vi "Modulo_Triggers.vi"(0 "Motion Settings In":T1={"No Motion?"=FALSE, "Motion System"=enum."NI 735x", "Motion Bd ID"=1, "Motion Profile"="SMAC1", "# Axis"=1, "Reverse Z axis?"=TRUE, "SMAC Axis"=0, "scan pair"=enum."y-(x) scan", "RT fps"=6.0, "Steps per mm"=[1000, 1000, 1000, 1000], "Motor Parameters"={"velocity ct/s"=[10000.0, 10000.0, 10000.0, 50000.0], "accel ct/s^2"=[50000.0, 50000.0, 50000.0, 200000.0]}, "One Way Scan"=FALSE, "Reverse One Way Scan"=FALSE, "Global Position (mm)"=[], "Plane"=0, "Distance between\nscan lines (um)"=0.0, "Distance between\nscan planes (um)"=0.0, "number of scan planes"=1, "Total steps in line"=0, "Xtra plane\ndistance  (um)"=100, "Xtra planes "=1, "Add Axis"=FALSE, "overshoot cts"=200, "BKPT Shift"=0, "Scan Start Time (ms)"=0, "ESP VISA"="GPIB::1::INSTR", "3rd Axis"=1, "GL Ref Out"=refnum, "Galil Address"=""} {"3rd Axis" items=["x", "y", "z", "w"]; "Xtra planes" min=1; "Xtra plane\ndistance  (um)" min=0; "Distance between\nscan planes (um)" format="%.2f"; "Distance between\nscan lines (um)" format="%.2f"; "SMAC Axis" items=["None"=0, "Axis 1"=1, "Axis 2"=2, "Axis 3"=3, "Axis 4"=4, "Axis 5"=5, "Axis 6"=6, "Axis 7"=7, "Axis 8"=8, "Vector Space 1"=17, "Vector Space 2"=18, "Vector Space 3"=19, "Vector Space 4"=20]; "Motion Bd ID" min=1 max=32 step=1}, 1 "Axis":u16(ring)=1 items=["Axis 1"=1, "Axis 2"=2, "Axis 3"=3, "Axis 4"=4, "Axis 5"=5, "Axis 6"=6, "Axis 7"=7, "Axis 8"=8], 2 "Reverse ?":bool, 5 "Program (1)":u8=4 format="%.0x", 11 "error in (no error)":errorcluster, 13 "Offset":i32) -> (4 "Start Position":i32, 15 "error out":errorcluster)   [LabVIEW 2022 SP3]
doc: "EXAMPLE: DO_WHILE Loop (Onboard Programming Template)\n\nSUMMARY:\nThis FlexMotion example demonstrates the implementation of a DO_WHILE loop data structure in an onboard program. The C equivalent of the data structure implemented here is:\n\ndo {\n// code to be repeated\nloopVar = loopVar - increment;\n} while (loopVar != 0);\n\nTHEORY OF OPERATION:\nThe flow of the DO_WHILE loop data structure goes as follows:\n(1) Program storage is begun.\n(2) The DO_WHILE loop is set up. (Loop Variable and Increment are each defined and initialized.)\n(3) A code delimiter is set using label #1.\n(4) Code to be executed each time through loop is run (in the template program, the loop variable is decremented).\n(5) The loop variable or other test condition is checked.\n(6) If the test condition is true, then we jump back to label #1. Otherwise, the condition is false so the loop terminates.\n(7) Program storage is ended.\n\nDEVELOPMENT DETAILS:\nApplication Software: LabVIEW 5.0.x\nHardware: FlexMotion controller\nDriver Software: FlexMotion Software 4.0\n\nREQUIRED HARDWARE:\n(controller only)\n\nINSTRUCTIONS:\n(0) Initialize the FlexMotion controller before running this VI. \n(1) Add the FlexMotion functions you want to execute into the block diagram where noted.\n(2) Run the VI to store the program. (The program will not be executed at this time.)\n(3) You can then run the program you have stored by calling the run_prog.flx function with the appropriate program number.\n\nADDITIONAL NOTES:\n(a) You should read the following items before writing FlexMotion onboard programs:\n(1) The Onboard Programs section of the FlexMotion Hardware User Manual (page 4-9 in the November 1998 edition).\n(2) The section about onboard variables in your FlexMotion Software Reference Manual (pages 4-11 and 4-12 in the November 1998 edition)\n(3) You will find the chapter of the FlexMotion Software Reference Manual concerning the Onboard Programming functions to be an invaluable reference resource (Chapter 12 of the November 1998 edition) along with the online help for the VI functions.\n(b) This template repeats the DO_WHILE loop as long as an expression with a variable evaluates to be true. However, you may evaluate other conditions such as move complete status instead.\n\n*NOTE: This example is not supported on the 7334 controller."
uses:
  MotionParameters.ctl
  MotionSys.ctl
  -MotionRoutines/ScanAxis.ctl
  -MotionRoutines/3rdAxis.ctl
  <vilib>/Motion/FlexMotion/FunctionsVIs/StartStopMotion.llb/Start Motion (8 axes).flx
  <vilib>/Motion/FlexMotion/FunctionsVIs/Trajectory.llb/Load Acceleration/Deceleration.flx
  <vilib>/Motion/FlexMotion/FunctionsVIs/OnboardProgramming.llb/Jump to Label on Condition (8 axes).flx
  <vilib>/Motion/FlexMotion/FunctionsVIs/OnboardProgramming.llb/Wait on Condition (8 axes).flx
panel:
  out "Store Loop":i32
  # "This will only work with735X controllers"
  # "1-D and 2-D B scan settings"
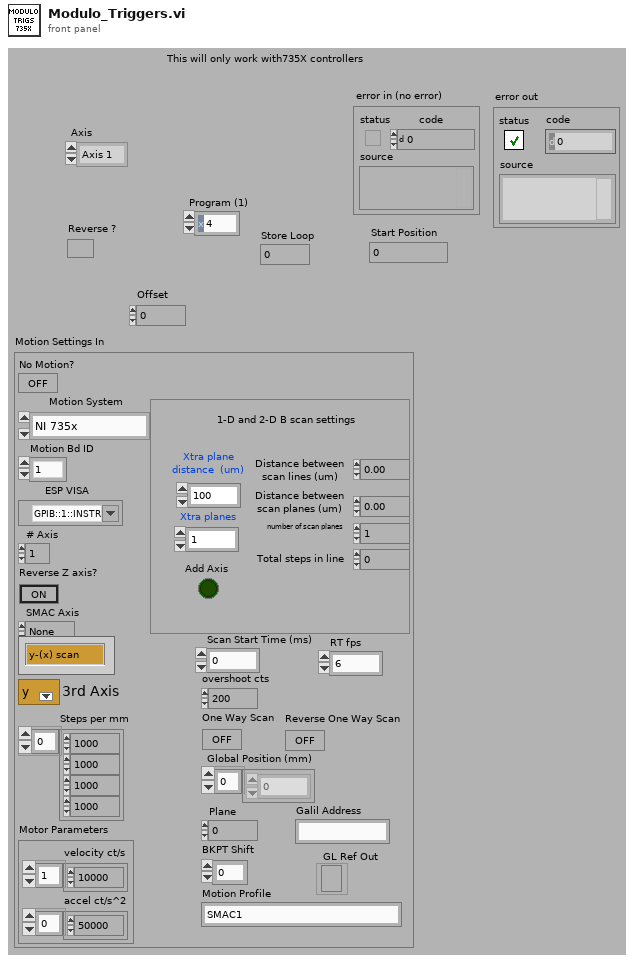
[diagram p1: front panel]
types:
  T1 = typedef "MotionParameters.ctl" = cluster{"No Motion?":bool, "Motion System":T2, "Motion Bd ID":u8, "Motion Profile":string, "# Axis":i8, "Reverse Z axis?":bool, "SMAC Axis":u16, "scan pair":T3, "RT fps":sgl, "Steps per mm":i32[], "Motor Parameters":cluster{"velocity ct/s":dbl[], "accel ct/s^2":dbl[]}, "One Way Scan":bool, "Reverse One Way Scan":bool, "Global Position (mm)":dbl[], "Plane":i32, "Distance between\nscan lines (um)":sgl, "Distance between\nscan planes (um)":sgl, "number of scan planes":i32, "Total steps in line":i32, "Xtra plane\ndistance  (um)":i32, "Xtra planes ":i32, "Add Axis":bool, "overshoot cts":i32, "BKPT Shift":i32, "Scan Start Time (ms)":u32, "ESP VISA":refnum<visa-resource-name>, "3rd Axis":T4, "GL Ref Out":refnum<k7>, "Galil Address":string}
  T2 = typedef "MotionSys.ctl" = enum16{"MM3000", "NI 735x", "Newport ESP", "No Motion Card", "Galil"}
  T3 = typedef "ScanAxis.ctl" = enum16{"y-(x) scan", "x-(y) scan", "z-(x) scan", "z-(y) scan", "y-(z) scan", "x-(z) scan", "w-(x) scan", "w-(y) scan", "w-(z) scan", "x-(w) scan", "y-(w) scan", "z-(w) scan"}
  T4 = typedef "3rdAxis.ctl" = u16
  T5 = enum16{"No Change", "Reset on Breakpoint", "Set on Breakpoint", "Toggle on Breakpoint", "Create Pulse on Breakpoint"}
  T6 = enum16{"Absolute Breakpoint", "Relative Breakpoint", "Modulo Breakpoint", "Periodic Breakpoint"}
  T7 = typedef "Var" = u8
  T8 = enum16{"Less Than", "Equal", "Less Than Or Equal", "Greater Than", "Not Equal", "Greater Than Or Equal", "True", "Home Found", "Index Found", "High Speed Capture", "Position Breakpoint", "Reserved", "Velocity Threshold", "Move Complete", "Profile Complete", "Blend Complete", "Motor Off", "Home Input Active", "Limit Input Active", "Software Limit Active", "Program Complete", "IO Port Match"}
  T9 = typedef "Bd Id Out" = u8
  T10 = typedef "Resource Out (Enum).flx" = u16
  T11 = typedef "Resource Out.flx" = u8
  T12 = cluster{"0":bool, "1":bool, "2":bool, "3":bool, "4":bool, "5":bool, "6":bool, "7":bool, "8":bool}
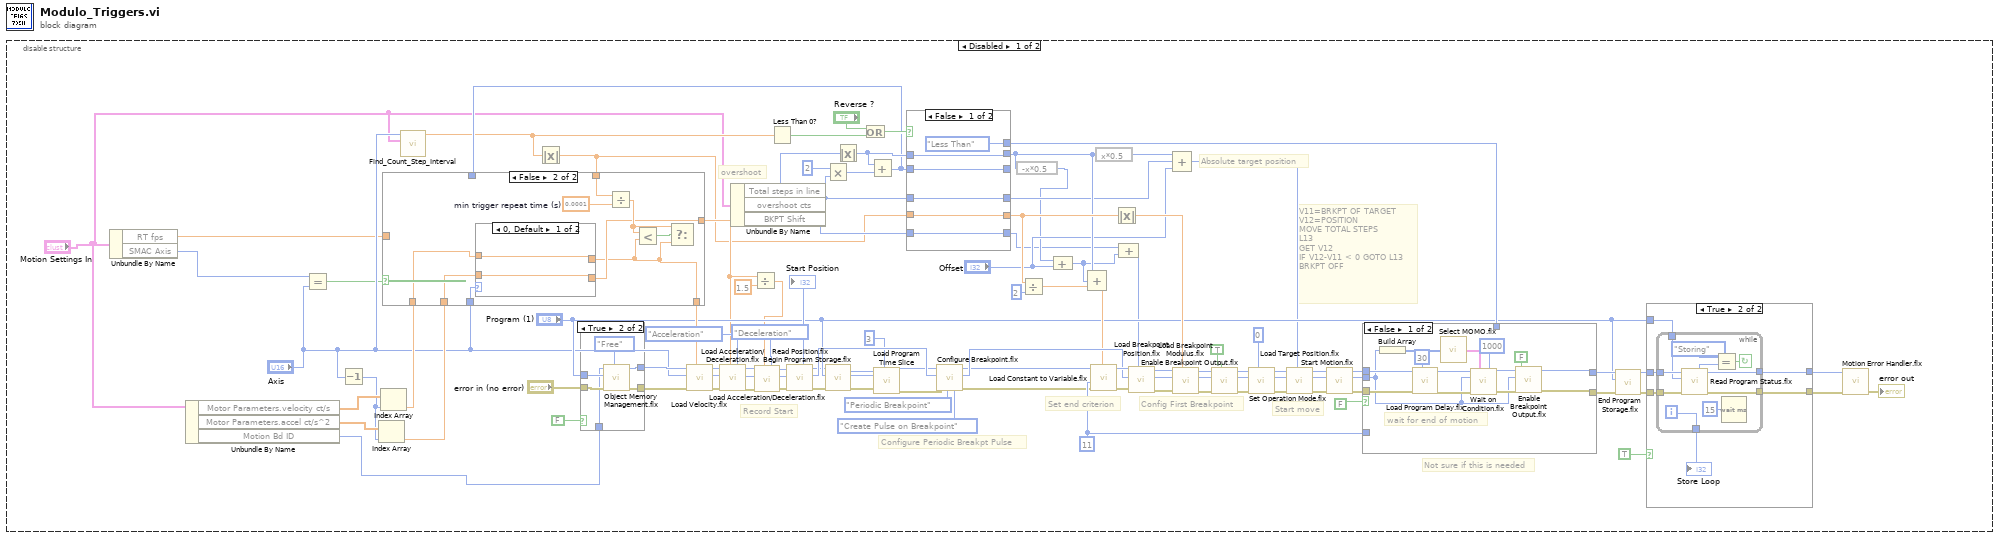
[diagram p0: block diagram]
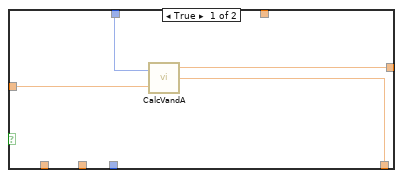
[diagram p4: hidden frame]
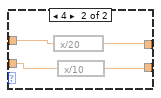
[diagram p5: hidden frame]
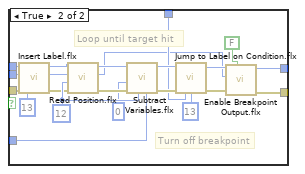
[diagram p6: hidden frame]
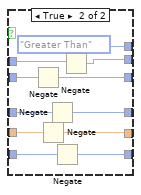
[diagram p7: hidden frame]
diagram:
  n1 = disable-structure shown="Disabled" {
    frame Disabled {
      w105 = T7 11 ("Step Int Variable")
      # "Absolute target position"
      # "Not sure if this is needed"
      # "Configure Periodic Breakpt Pulse"
      # "Set end criterion"
      # "overshoot"
      # "V11=BRKPT OF TARGET\nV12=POSITION\nMOVE TOTAL STEPS\nL13\nGET V12\nIF V12-V11 < 0 GOTO L13\nBRKPT OFF"
      # "Record Start"
      # "Config First Breakpoint"
      # "Start move"
      n2 = Unbundle By Name("Motion Settings In") -> ("RT fps"=w6:sgl, "SMAC Axis"=w9:u16)
      n3 = Unbundle By Name("Motion Settings In") -> ("Motor Parameters.velocity ct/s"=w16:dbl[], "Motor Parameters.accel ct/s^2"=w15:dbl[], "Motion Bd ID"=w1:u8)
      n4 = Equal?(x=w9, y="Axis") -> (x = y?=w2:bool)
      n5 = Decrement(x="Axis") -> (x-1=w11:u16)
      n6 = Index Array(array=w15, index=w11) -> (element=w13:dbl)
      n7 = Index Array(array=w16, index=w11) -> (element=w14:dbl)
      n8 = call "Find_Count_Step_Interval.vi"("Motion Settings In"="Motion Settings In", "Axis"="Axis") -> ("BP Interval"=w12:dbl)  [unwired: 8 in, 1 out]
      n9 = Absolute Value(x=w12) -> (abs(x)=w3:dbl)
      n10 = case shown="True" FALSE {
        tunnel: "error in (no error)" -> [w107 w112]
        tunnel: "Program (1)" -> [_ w111]
        tunnel: [w106 w110] -> w44
        tunnel: [w107 w109] -> w43
        tunnel: w1 -> [w106 w108]
        frame False {
        }
        frame True {
          n11 = call <vilib>:"Object Memory Management.flx"("Operation"=enum16{"Save", "Delete", "Free"}."Free" ("Operation (Free)"), "error in (no error)"=w112, "Object (1)"=w111, "Board ID"=w108) -> ("error out"=w109:errorcluster, "Bd ID Out"=w110:T9)  [unwired: 4 out]
        }
      }
      n12 = Unbundle By Name("Motion Settings In") -> ("Total steps in line"=w5:i32, "overshoot cts"=w7:i32, "BKPT Shift"=w4:i32)
      n13 = Less Than 0?(x=w12) -> (x < 0?=w94:bool)
      n14 = Multiply(x=2, y=w7) -> (x*y=w58:i32)
      n15 = Absolute Value(x=w5) -> (abs(x)=w64:i32)
      n16 = Or(x="Reverse ?", y=w94) -> (x .or. y?=w92:bool)
      n17 = Add(x=w64, y=w58) -> (x+y=w57:i32)
      n18 = case shown="False" w2 {
        tunnel: [w132 w140] -> w27
        tunnel: [w133 w136] -> w80
        tunnel: w3 -> [_ w141]
        tunnel: w57 -> [w135 _]
        tunnel: w6 -> [w134 _]
        tunnel: "Axis" -> [_ w139]
        tunnel: w14 -> [_ w138]
        tunnel: w13 -> [_ w137]
        frame True {
          n19 = call "CalcVandA.vi"("distance"=w135, "fps"=w134) -> ("Accel"=w132:dbl, "Velocity"=w133:dbl)  [unwired: 1 out]
        }
        frame False {
          w142 = 0.0001  # min trigger repeat time (s)
          n20 = case shown="0, Default" w139 {
            tunnel: w138 -> [w146 w150]
            tunnel: w137 -> [w145 w147]
            tunnel: [w146 w149] -> w136
            tunnel: [w145 w148] -> w140
            frame 0, Default {
            }
            frame 4 {
              n21 = expression code="x/20"(w150) -> (w149:dbl)
              n22 = expression code="x/10"(w147) -> (w148:dbl)
            }
          }
          n23 = Divide(x=w141, y=w142) -> (x/y=w143:dbl)
          n24 = Less?(x=w143, y=w136) -> (x < y?=w144:bool)
          n25 = Select(t=w143, s=w144, f=w136) -> ()  [unwired: 1 out]
        }
      }
      n26 = call <vilib>:"Load Velocity.flx"("Velocity (10000)"=w80, "error in (no error)"=w43, "Axis or Vector Space"="Axis", "Board ID"=w44) -> ("error out"=w91:errorcluster, "Resource Output"=w89:T10, "Bd ID Out"=w90:T9)  [unwired: 3 out]
      n27 = call "Load Acceleration/Deceleration.flx"("Acceleration Type (Both)"=enum16{"Both", "Acceleration", "Deceleration"}."Acceleration", "Acceleration (100000)"=w27, "error in (no error)"=w91, "Axis or Vector Space"=w89, "Board ID"=w90) -> ("error out"=w32:errorcluster, "Resource Output"=w31:T10, "Bd ID Out"=w35:T9)  [unwired: 2 out]
      n28 = Divide(x=w27, y=1.5) -> (x/y=w26:dbl)
      n29 = call "Load Acceleration/Deceleration.flx"("Acceleration Type (Both)"=enum16{"Both", "Acceleration", "Deceleration"}."Deceleration", "Acceleration (100000)"=w26, "error in (no error)"=w32, "Axis or Vector Space"=w31, "Board ID"=w35) -> ("error out"=w33:errorcluster, "Resource Output"=w30:T10, "Bd ID Out"=w34:T9)  [unwired: 2 out]
      n30 = call <vilib>:"Read Position.flx"("error in (no error)"=w33, "Axis"=w30, "Board ID"=w34) -> ("error out"=w52:errorcluster, "Resource Output"=w65:T10, "Bd ID Out"=w53:T9, "Position"=→"Start Position":i32)  [unwired: 3 out]
      n31 = call <vilib>:"Begin Program Storage.flx"("error in (no error)"=w52, "Program (1)"="Program (1)", "Board ID"=w53) -> ("error out"=w42:errorcluster, "Resource Out"=w37:T11, "Bd ID Out"=w39:T9)  [unwired: 3 out]
      n32 = call <vilib>:"Load Program Time Slice.vi"("Time Slice (ms)"=u32 3, "error in (no error)"=w42, "Program"=w37, "Board ID"=w39) -> ("error out"=w41:errorcluster, "Bd ID Out"=w40:T9)  [unwired: 1 in, 2 out]
      n33 = case shown="False" w92 {
        tunnel: w57 -> [w191 w202]
        tunnel: [w191 w201] -> _
        tunnel: [T8."Less Than" ("Condition Code (True)") T8."Greater Than" ("Condition Code (True)")] -> w95
        tunnel: [w189 w198] -> w47
        tunnel: w7 -> [w189 w199]
        tunnel: w3 -> [w188 w197]
        tunnel: [w188 w196] -> w76
        tunnel: [w187 w194] -> w49
        tunnel: w64 -> [w187 w195]
        tunnel: w4 -> [w186 w193]
        tunnel: [w186 w192] -> w23
        frame False {
        }
        frame True {
          n34 = Negate(x=w202) -> (-x=w201:i32)
          n35 = Negate(x=w197) -> (-x=w196:dbl)
          n36 = Negate(x=w199) -> (-x=w198:i32)
          n37 = Negate(x=w193) -> (-x=w192:i32)
          n38 = Negate(x=w195) -> (-x=w194:i32)
        }
      }
      n39 = call <vilib>:"Configure Breakpoint.flx"("Action (No Change)"=T5."Create Pulse on Breakpoint", "Mode (Absolute)"=T6."Periodic Breakpoint", "error in (no error)"=w41, "Axis or Encoder"=w65, "Board ID"=w40) -> ("error out"=w51:errorcluster, "Resource Output"=w75:T10, "Bd ID Out"=w50:T9)  [unwired: 1 in, 3 out]
      n40 = expression code="-x*0.5"(w49) -> (w25:i32)
      n41 = Divide(x=w76, y=2) -> (x/y=w63:dbl)
      n42 = Compound Arithmetic op=ADD(w25, "Offset") -> (w24:i32)
      n43 = Compound Arithmetic op=ADD(w49, w24, w63) -> (w62:dbl)
      n44 = call <vilib>:"Load Constant to Variable.flx"("Value (0)"=w62, "error in (no error)"=w51, "Var"=w105, "Board ID"=w50) -> ("error out"=w85:errorcluster, "Bd ID Out"=w86:T9)  [unwired: 4 out]
      n45 = expression code="x*0.5"(w49) -> (w48:i32)
      n46 = Absolute Value(x=w76) -> (abs(x)=w61:dbl)
      n47 = Compound Arithmetic op=ADD(w23, w24) -> (w22:i32)
      n48 = call <vilib>:"Load Breakpoint Position.flx"("Breakpoint Position (0)"=w22, "error in (no error)"=w85, "Axis or Encoder"=w75, "Board ID"=w86) -> ("error out"=w83:errorcluster, "Resource Output"=w82:T10, "Bd ID Out"=w84:T9)  [unwired: 3 out]
      n49 = Compound Arithmetic op=ADD(w48, w47, "Offset") -> (w45:i32)
      n50 = call <vilib>:"Load Breakpoint Modulus.flx"("Breakpoint Modulus (0)"=w61, "error in (no error)"=w83, "Axis or Encoder"=w82, "Board ID"=w84) -> ("error out"=w69:errorcluster, "Resource Output"=w70:T10, "Bd ID Out"=w71:T9)  [unwired: 3 out]
      n51 = call <vilib>:"Enable Breakpoint Output.flx"("Enable Breakpoint"=TRUE, "error in (no error)"=w69, "Axis or Encoder"=w70, "Board ID"=w71) -> ("error out"=w68:errorcluster, "Resource Output"=w66:T10, "Bd ID Out"=w67:T9)  [unwired: 3 out]
      n52 = call <vilib>:"Set Operation Mode.flx"("Position Mode (Absolute)"=0, "error in (no error)"=w68, "Axis or Vector Space"=w66, "Board ID"=w67) -> ("error out"=w101:errorcluster, "Resource Output"=w98:T10, "Bd ID Out"=w102:T9)  [unwired: 2 out]
      n53 = call <vilib>:"Load Target Position.flx"("Target Position (0)"=w45, "error in (no error)"=w101, "Axis"=w98, "Board ID"=w102) -> ("error out"=w103:errorcluster, "Resource Output"=w104:T10, "Bd ID Out"=w99:T9)  [unwired: 3 out]
      n54 = call-poly <vilib>:"Start Motion.flx"("error in (no error)"=w103, "Axis or Vector Space"=w104, "Board ID"=w99) -> ("error out"=w78:errorcluster, "Resource Output"=w56:T10, "Bd ID Out"=w79:T9)  [unwired: 1 in, 2 out]
      n55 = case shown="False" FALSE ("Case Constant\n(See Context Help)") {
        tunnel: w105 -> [_ w182]
        tunnel: w95 -> [_ w175]
        tunnel: w79 -> [w159 w174]
        tunnel: w78 -> [w156 w173]
        tunnel: [w153 w169] -> w77
        tunnel: w56 -> [w151 w165]
        tunnel: [w154 w170] -> w55
        frame False {
          # "wait for end of motion"
          n56 = Build Array(w151) -> (w163:T10[])
          n57 = call <vilib>:"Load Program Delay.flx"("Delay Value (1 ms)"=30, "error in (no error)"=w156, "Board ID"=w159) -> ("error out"=w157:errorcluster, "Bd ID Out"=w158:T9)  [unwired: 4 out]
          n58 = call <vilib>:"Select MOMO.flx"("Resource"=w163) -> ("Must On/Off"=w164:T12)
          n59 = call-poly <vilib>:"Wait on Condition.flx"("Board ID"=w158, "Must On (False)"=w164, "Timeout (1)"=u16 1000, "Resource (0)"=w151, "error in (no error)"=w157) -> ("Bd ID Out"=w161:T9, "error out"=w160:errorcluster)  [unwired: 4 in, 5 out]
          n60 = call <vilib>:"Enable Breakpoint Output.flx"("Enable Breakpoint"=FALSE, "error in (no error)"=w160, "Axis or Encoder"=w151, "Board ID"=w161) -> ("error out"=w153:errorcluster, "Bd ID Out"=w154:T9)  [unwired: 4 out]
        }
        frame True {
          w183 = T7 12 ("Position Variable")
          # "Turn off breakpoint"
          # "Loop until target hit"
          n61 = call <vilib>:"Insert Label.flx"("Label Number (1)"=u16 13 ("Label"), "error in (no error)"=w173, "Board ID"=w174) -> ("error out"=w180:errorcluster, "Bd ID Out"=w181:T9)  [unwired: 4 out]
          n62 = call <vilib>:"Read Position.flx"("error in (no error)"=w180, "Retn Vect"=w183, "Axis"=w165, "Board ID"=w181) -> ("error out"=w178:errorcluster, "Resource Output"=w167:T10, "Bd ID Out"=w179:T9)  [unwired: 3 out]
          n63 = call <vilib>:"Subtract Variables.flx"("Var 2"=w182, "Var 1"=w183, "error in (no error)"=w178, "Ret Vect"=T7 0 ("Position Variable"), "Board ID"=w179) -> ("error out"=w176:errorcluster, "Bd ID Out"=w177:T9)  [unwired: 3 out]
          n64 = call-poly <vilib>:"Jump to Label on Condition.flx"("Board ID"=w177, "error in (no error)"=w176, "Condition Code (True)"=w175, "Jump to Label (1)"=u16 13) -> ("Bd ID Out"=w172:T9, "error out"=w171:errorcluster)  [unwired: 4 in, 6 out]
          n65 = call <vilib>:"Enable Breakpoint Output.flx"("Enable Breakpoint"=FALSE, "error in (no error)"=w171, "Axis or Encoder"=w167, "Board ID"=w172) -> ("error out"=w169:errorcluster, "Bd ID Out"=w170:T9)  [unwired: 4 out]
        }
      }
      n66 = call <vilib>:"End Program Storage.flx"("error in (no error)"=w77, "Program (1)"="Program (1)", "Board ID"=w55) -> ("error out"=w96:errorcluster, "Bd ID Out"=w97:T9)  [unwired: 4 out]
      n67 = case shown="True" TRUE {
        tunnel: w97 -> [w115 w121]
        tunnel: w96 -> [w114 w120]
        tunnel: "Program (1)" -> [_ w119]
        tunnel: [w115 w117] -> w21
        tunnel: [w114 w116] -> w20
        frame False {
        }
        frame True {
          n68 = while {
            tunnel: w121 -> [w131]
            tunnel: w120 -> [w130]
            tunnel: [w129] -> w117
            tunnel: [w128] -> w116
            tunnel: w119 -> [w127]
            tunnel: [w123] -> w118
            i -> [w123]
            stop <- w124 continue-if-true
            n69 = call <vilib>:"Read Program Status.flx"("error in (no error)"=w130, "Program (1)"=w127, "Board Id"=w131) -> ("error out"=w128:errorcluster, "Bd Id Out"=w129:T9, "Program Status"=w125:enum16{"Done", "Playing", "Paused", "Storing"})  [unwired: 4 out]
            n70 = Equal?(x=enum16{"Done", "Playing", "Paused", "Storing"}."Storing" ("Program Status"), y=w125) -> (x = y?=w124:bool)
            n71 = Wait (ms)(milliseconds to wait=15) -> ()  [unwired: 1 out]
          }
          "Store Loop" <- w118
        }
      }
      n72 = call <vilib>:"Motion Error Handler.flx"("Board ID"=w21, "error in (no error)"=w20) -> ("error out"=→"error out":errorcluster)  [unwired: 4 in, 9 out]
    }
    frame Enabled {
    }
  }
